vi "全局.vi"() -> ()   [LabVIEW 2015]
panel:
  out "重测温度":string
  out "行号":i32
  in  "测量通道数":i32=2
  in  "暂停":bool
  in  "温度表格":string[][](table)
  in  "编号表格":string[][](table)
  in  "停止":bool
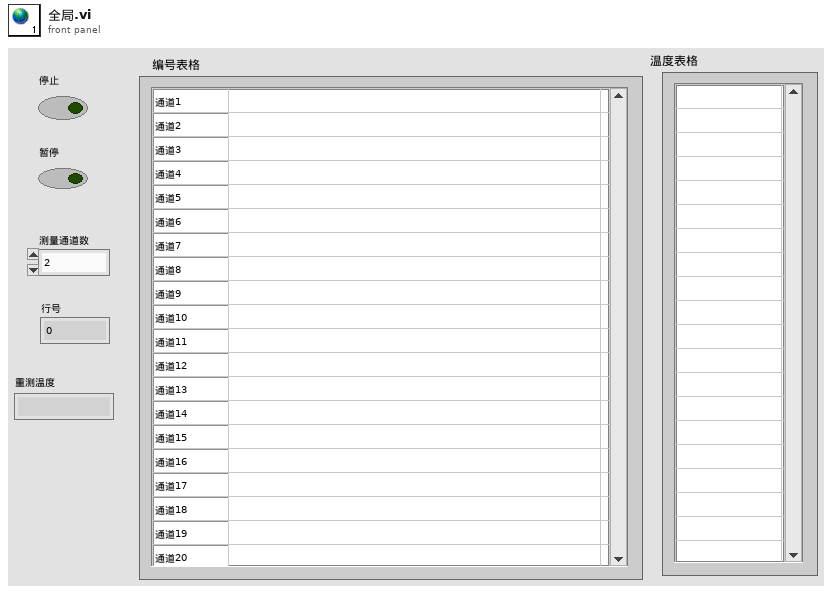
[diagram p1: front panel]
diagram:
